vi "RobotMainVI_RefNum_Simulation_Global.vi"(0 "menu":enum16{"set", "get", "delete"}(ring)=enum."get", 7 "VI Refnum in":refnum<vi>, 11 "error in (no error)":errorcluster) -> (8 "VI Refnum out":refnum<vi>, 15 "error out":errorcluster)   [LabVIEW 2017]
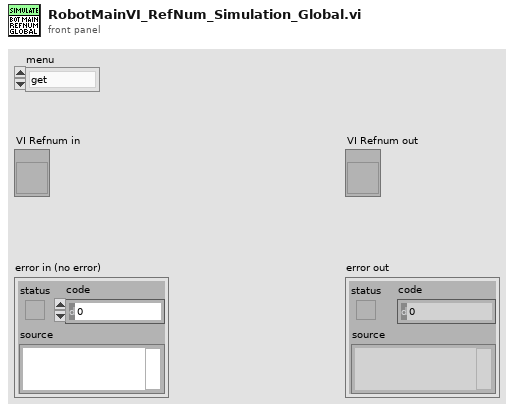
[diagram p1: front panel]
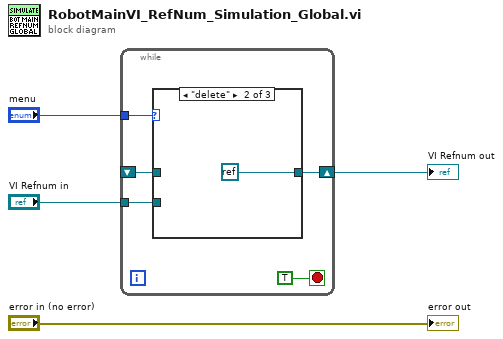
[diagram p0: block diagram]
diagram:
  n1 = while {
    tunnel: "menu" -> [w8]
    shift-right: [w6] -> w1
    shift-left: _ -> [w7]
    tunnel: "VI Refnum in" -> [w5]
    stop <- TRUE stop-if-true
    n2 = case shown="\"delete\"" w8 {
      tunnel: w7 -> [_ _ w12]
      tunnel: [w10 refnum<k0> refnum w12] -> w6
      tunnel: w5 -> [w10 _ _]
      frame "set" {
      }
      frame "delete" {
      }
      frame "get", Default {
      }
    }
  }
  "VI Refnum out" <- w1
  "error out" <- "error in (no error)"
